vi "Draw Picture.vi"(10 "picture in":picture, 11 "Game Componants in":refnum<class "Game Componants.lvclass">) -> (2 "picture out":picture)   [LabVIEW 2021, in "Game Componants.lvclass"]
doc: "MIT Licence\nCopyright (c) 2024 David Grollier"
uses:
  Game Componants.lvclass
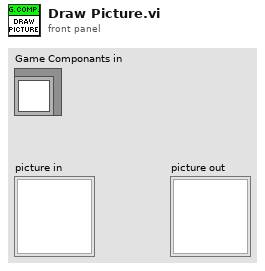
[diagram p1: front panel]
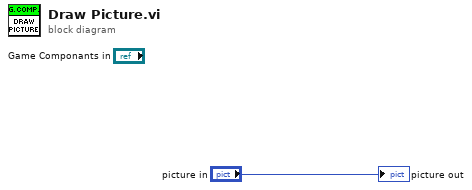
[diagram p0: block diagram]
diagram:
  "picture out" <- "picture in"
